vi "Old - Turn Precise.vi"(6 "Angle Reduction Factor":dbl, 8 "error in (no error)":errorcluster, 10 "Ref-Nums":T1, 11 "Angle":dbl) -> (0 "error out":errorcluster)   [LabVIEW 2016]
uses:
  <vilib>/Rock Robotics/WPI/Utilities/WPI_GetSetVariantRefNum.vi
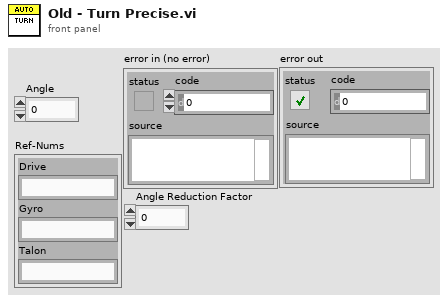
[diagram p1: front panel]
types:
  T1 = cluster{"Drive":string, "Gyro":string, "Talon":string}
  T2 = typedef "WPI_GyroDevRef.ctl" = cluster{"DevStatus":errorcluster, "Analog Channel":T3, "Offset":dbl, "Gain (VoltsPerDegree/Second)":dbl, "Gyro Type":enum16{"Analog", "XRS450"}, "Handle":i32, "SPI Bus":T4, "Device Found":bool, "Sample Rate":dbl, "Calibrate On Open":bool}
  T3 = typedef "FPGA_AIChannel.ctl" = enum8{"AI 0", "AI 1", "AI 2", "AI 3", "AI MXP 0", "AI MXP 1", "AI MXP 2", "AI MXP 3", "Invalid"}
  T4 = typedef "spi_bus.ctl" = enum16{"SPI On-Board, CS0", "SPI On-Board, CS1", "SPI On-Board, CS2", "SPI On-Board, CS3", "SPI MXP", "Invalid"}
  T5 = typedef "WPI_RobotDriveDevRef.ctl" = cluster{"DevStatus":errorcluster, "Motors[]":T6[], "Square Inputs":bool, "Max Output":dbl}
  T6 = typedef "WPI_MotorControlDeviceRef.ctl" = cluster{"DeviceStatus":errorcluster, "Type":T7, "PWM":cluster{"PWM Channel":T8, "DeadBand":T9}, "CAN":cluster{"Device Number":u8, "SetOutput VI Ref":variant, "GetOutput VI Ref":variant, "Enable VI Ref":variant, "Disable VI Ref":variant, "Data":variant}, "Invert":bool}
  T7 = typedef "WPI_MotorControlType.ctl" = enum16{"PWM", "CAN"}
  T8 = typedef "FPGA_DIOPWMChannel.ctl" = enum8{"PWM 0", "PWM 1", "PWM 2", "PWM 3", "PWM 4", "PWM 5", "PWM 6", "PWM 7", "PWM 8", "PWM 9", "PWM MXP 0", "PWM MXP 1", "PWM MXP 2", "PWM MXP 3", "PWM MXP 4", "PWM MXP 5", "PWM MXP 6", "PWM MXP 7", "PWM MXP 8", "PWM MXP 9", "Invalid"}
  T9 = typedef "WPI_PWMDeadband.ctl" = cluster{"Name":string, "maxPositivePwm":i32, "minPositivePwm":i32, "centerPwm":i32, "maxNegativePwm":i32, "minNegativePwm":i32, "angularRange":u16}
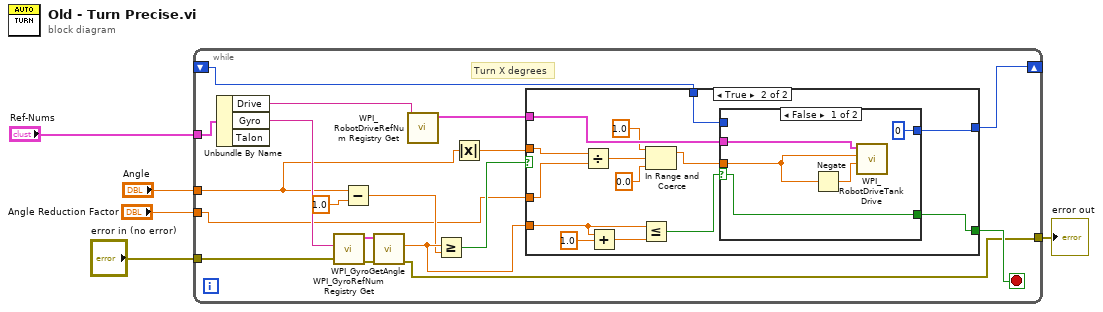
[diagram p0: block diagram]
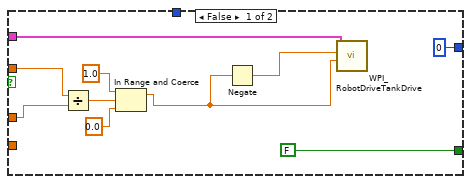
[diagram p2: hidden frame]
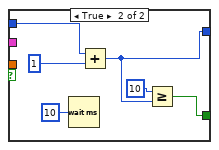
[diagram p3: hidden frame]
diagram:
  n1 = while {
    tunnel: "Angle" -> [w6]
    tunnel: "Ref-Nums" -> [w16]
    shift-right: [w13] -> _
    shift-left: _ -> [w12]
    tunnel: "error in (no error)" -> [w11]
    tunnel: [w10] -> w2
    tunnel: "Angle Reduction Factor" -> [w8]
    stop <- w18 stop-if-true
    # "Turn X degrees"
    n2 = Unbundle By Name(w16) -> ("Drive"=w15:string, "Gyro"=w14:string)  [unwired: 1 out]
    n3 = call <vilib>:"WPI_GyroRefNum Registry Get.vi"("error in (no error)"=w11, "refnum name"=w14) -> ("error out"=w22:errorcluster, "GyroDevRef"=w23:T2)  [unwired: 8 in]
    n4 = Subtract(x=w6, y=1.0) -> (x-y=w9:dbl)
    n5 = call <vilib>:"WPI_GyroGetAngle.vi"("error in"=w22, "GyroDevRef"=w23) -> ("error out"=w10:errorcluster, "Angle"=w19:dbl)  [unwired: 5 in, 3 out]
    n6 = call <vilib>:"WPI_RobotDriveRefNum Registry Get.vi"("refnum name"=w15) -> ("RobotDriveDevRef"=w20:T5)  [unwired: 9 in, 1 out]
    n7 = Greater Or Equal?(x=w19, y=w9) -> (x >= y?=w21:bool)
    n8 = Absolute Value(x=w6) -> (abs(x)=w7:dbl)
    n9 = case shown="True" w21 {
      tunnel: w20 -> [w33 w42]
      tunnel: w19 -> [_ w46]
      tunnel: [FALSE w44] -> w18
      tunnel: [0 w41] -> w13
      tunnel: w12 -> [_ w40]
      tunnel: w7 -> [w30 w38]
      tunnel: w8 -> [w29 w39]
      frame False {
        n10 = Divide(x=w30, y=w29) -> (x/y=w26:dbl)
        n11 = In Range and Coerce(upper limit=1.0 ("x"), x=w26, lower limit=0.0) -> (coerced(x)=w27:dbl)  [unwired: 1 out]
        n12 = Negate(x=w27) -> (-x=w28:dbl)
        n13 = call <vilib>:"WPI_RobotDriveTankDrive.vi"("Right axis value"=w27, "Left axis value"=w28, "RobotDriveDevRef"=w33) -> ()  [unwired: 6 in, 3 out]
      }
      frame True {
        n14 = Divide(x=w38, y=w39) -> (x/y=w35:dbl)
        n15 = Add(x=w46, y=1.0) -> (x+y=w47:dbl)
        n16 = Less Or Equal?(x=w46, y=w47) -> (x <= y?=w43:bool)
        n17 = In Range and Coerce(upper limit=1.0 ("x"), x=w35, lower limit=0.0) -> (coerced(x)=w34:dbl)  [unwired: 1 out]
        n18 = case shown="False" w43 {
          selector: w43 -> [w52 _]
          tunnel: [w52 w54] -> w44
          tunnel: w42 -> [w51 _]
          tunnel: w40 -> [_ w56]
          tunnel: [0 w55] -> w41
          tunnel: w34 -> [w48 _]
          frame False {
            n19 = Negate(x=w48) -> (-x=w49:dbl)
            n20 = call <vilib>:"WPI_RobotDriveTankDrive.vi"("Right axis value"=w49, "Left axis value"=w48, "RobotDriveDevRef"=w51) -> ()  [unwired: 6 in, 3 out]
          }
          frame True {
            n21 = Wait (ms)(milliseconds to wait=u32 10) -> ()  [unwired: 1 out]
            n22 = Add(x=w56, y=1) -> (x+y=w55:i32)
            n23 = Greater Or Equal?(x=10, y=w55) -> (x >= y?=w54:bool)
          }
        }
      }
    }
  }
  "error out" <- w2
